vi "Download_File.vi"(0 "File Contents":string, 1 "File Path Control":path, 2 "File Selection":u16(ring), 3 "Data":T1={"Info Box"="", "MAC & Name Out"=[], "Default Gateway"="", "Drfiter IP Addresses"=[], "Network Map"="", "Drifter Selection"=0, "File Selection"=0, "Download File Path"=path "", "File Selection Strings"=[], "Sample Rate"=enum." 0.2", "Log While Charging"=enum." Yes"}, 11 "Error In":errorcluster) -> (15 "Error Out":errorcluster)   [LabVIEW 2017]
uses:
  data.ctl
  <vilib>/Utility/file.llb/Write Delimited Spreadsheet (string).vi
panel:
  out "concatenated string":string
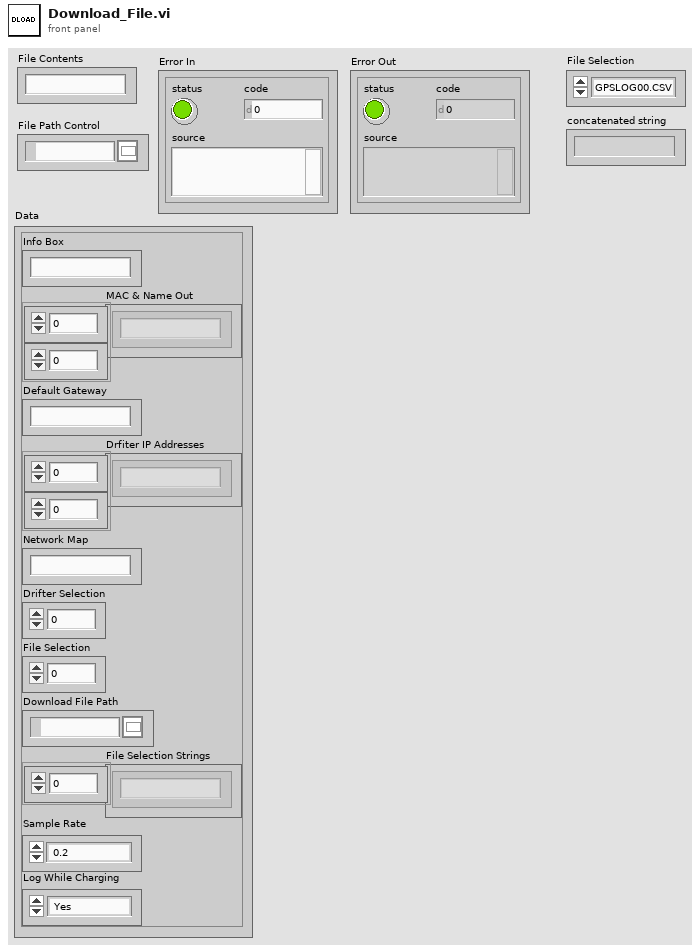
[diagram p1: front panel]
types:
  T1 = typedef "data.ctl" = cluster{"Info Box":string, "MAC & Name Out":string[][], "Default Gateway":string, "Drfiter IP Addresses":string[][], "Network Map":string, "Drifter Selection":i32, "File Selection":i32, "Download File Path":path, "File Selection Strings":string[], "Sample Rate":enum32{"No Selection", " 0.2", " 0.1", " 1", " 2", " 5", " 10"}, "Log While Charging":enum32{"No Selection", " Yes", " No"}}
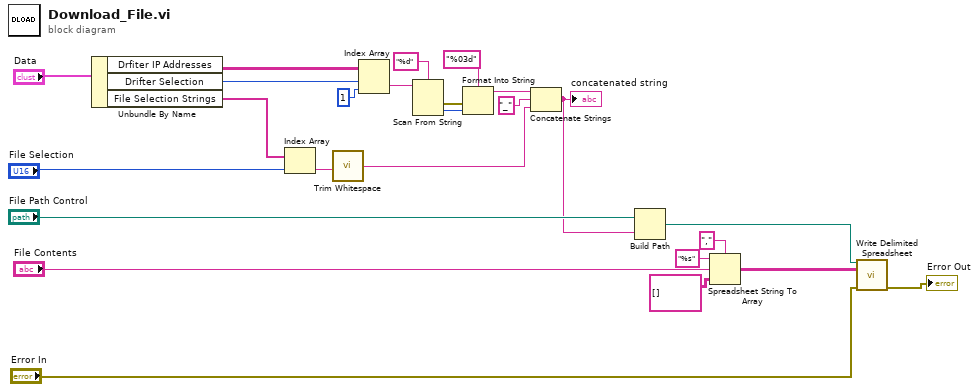
[diagram p0: block diagram]
diagram:
  n1 = Unbundle By Name("Data") -> ("Drfiter IP Addresses"=w23:string[][], "Drifter Selection"=w22:i32, "File Selection Strings"=w1:string[])
  n2 = Index Array(array=w1, index="File Selection") -> (element=w12:string)
  n3 = call <vilib>:"Trim Whitespace.vi"("string"=w12) -> ("trimmed string"=w11:string)  [unwired: 1 in]
  n4 = Index Array(array=w23, index (row)=w22, index (col)=1 ("disabled index (col)")) -> (element=w19:string)
  n5 = Scan From String(format string="%d", input string=w19) -> (error out=w17:errorcluster, output 1=w16:i32)  [unwired: 3 in, 2 out]
  n6 = Format Into String(format string="%03d", error in=w17, w16) -> (resulting string=w14:string)  [unwired: 1 in, 1 out]
  n7 = Concatenate Strings(w14, "_" ("string"), w11) -> (w10:string)
  "concatenated string" <- w10
  n8 = Build Path(base path="File Path Control", name or relative path=w10) -> (appended path=w4:path)
  n9 = Spreadsheet String To Array(delimiter (Tab)=",", format string="%s", spreadsheet string="File Contents", array type (2D Dbl)=string[][] []) -> (array=w5:string[][])
  n10 = call-poly <vilib>:"Write Delimited Spreadsheet.vi"("file path (dialog if empty)"=w4, "2D data"=w5, "error in (no error)"="Error In") -> ("error out"=→"Error Out":errorcluster)  [unwired: 11 in, 1 out]
